vi "Encode.vi"(8 "error in (no error)":errorcluster, 11 "ISO 15693 DOWN in":refnum<class "ISO 15693 DOWN.lvclass">) -> (0 "error out":errorcluster, 3 "ISO 15693 DOWN out":refnum<class "ISO 15693 DOWN.lvclass">)   [LabVIEW 2019, in "ISO 15693 DOWN.lvclass"]
uses:
  ISO 15693 DOWN.lvclass
  TypeDef/Store.ctl
  ISO 15693 DOWN.lvclass/ISO 15693 DOWN.ctl
  RFID system.lvclass
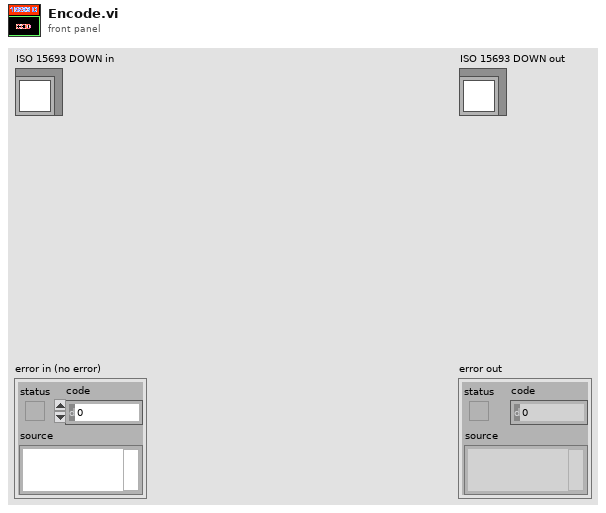
[diagram p1: front panel]
types:
  T1 = typedef "Store.ctl" = enum16{"envelope", "noise", "demSubCar", "CH_frame", "Decode", "demodulate", "in", "out", "sum", "subCarrier", "frame", "command", "encode", "modulate", "encode_UP", "modulate_up", "demod_up", "envelop_up", "sum_up", "out_up", "in_up"}
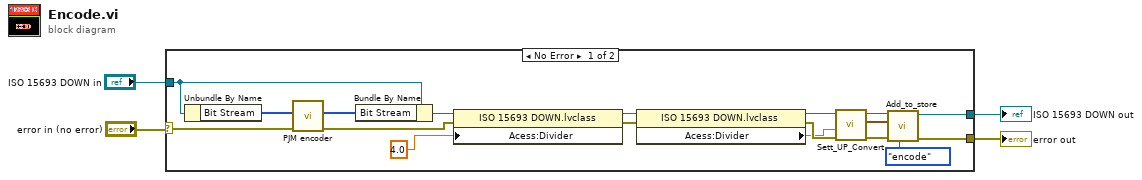
[diagram p0: block diagram]
diagram:
  n1 = case shown="No Error" "error in (no error)" {
    selector: "error in (no error)" -> [w21 w24]
    tunnel: [w14 w24] -> w3
    tunnel: "ISO 15693 DOWN in" -> [w20 w23]
    tunnel: [w13 w23] -> w1
    frame No Error {
      n2 = Unbundle By Name(w20) -> ("Bit Stream"=w22:u8[])
      n3 = call "PJM encoder.vi"("Error In"=w21, "Bit stream in"=w22) -> ("error out"=w9:errorcluster, "Bit stream out (1 from 4)"=w19:u8[])  [unwired: 8 in]
      n4 = Bundle By Name(cluster=w20, "Bit Stream"=w19) -> (w15:refnum<class "ISO 15693 DOWN.lvclass">)
      n5 = property class="ISO 15693 DOWN.lvclass"(reference=w15, error in=w9, "Acess:Divider"=4.0 ("Divider(1)")) -> (reference out=w11:refnum<class "ISO 15693 DOWN.lvclass">, error out=w8:errorcluster)
      n6 = property class="ISO 15693 DOWN.lvclass"(reference=w11, error in=w8) -> (reference out=w10:refnum<class "ISO 15693 DOWN.lvclass">, error out=w7:errorcluster, "Acess:Divider"=w5:dbl)
      n7 = call-dynamic "Sett_UP_Convert.vi"("error in (no error)"=w7, "Divider(1)"=w5, "ISO 15693 DOWN in"=w10) -> ("error out"=w16:errorcluster, "Waveform"=w17:waveform(dbl), "ISO 15693 DOWN out"=w18:refnum<class "ISO 15693 DOWN.lvclass">)  [unwired: 6 in]
      n8 = call "Add_to_store.vi"("Store"=Store."encode", "error in (no error)"=w16, "Waveform"=w17, "RFID system in"=w18) -> ("error out"=w14:errorcluster, "RFID system out"=w13:refnum<class "ISO 15693 DOWN.lvclass">)  [unwired: 6 in]
    }
    frame Error {
    }
  }
  "error out" <- w3
  "ISO 15693 DOWN out" <- w1
